vi "Authenticate.vi"(8 "error in (no error)":errorcluster, 10 "Authentication Inputs":T2, 11 "Authentication Provider in":refnum<class "Authentication Provider.lvclass">) -> (0 "error out":errorcluster, 2 "Authentication Outputs":T1, 3 "Authentication Provider out":refnum<class "Authentication Provider.lvclass">)   [LabVIEW 2020, in "HTTP Server.lvlib" / "Authentication Provider.lvclass"]
uses:
  Authentication Provider.lvclass
  Session/Session.lvclass
  lv-http-util/HTTP Utils/Request/Request.lvclass
  User Provider/User Provider.lvclass
  Authentication Inputs.ctl
  HTTP Server.lvlib
  User/User.lvclass
  Authentication Outputs.ctl
  Password Encoder/Password Encoder.lvclass
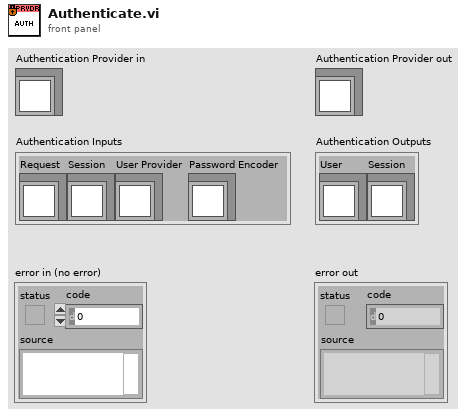
[diagram p1: front panel]
types:
  T1 = typedef "HTTP Server.lvlib/Authentication Outputs.ctl" = cluster{"User":refnum<class "User.lvclass">, "Session":refnum<class "Session.lvclass">}
  T2 = typedef "HTTP Server.lvlib/Authentication Inputs.ctl" = cluster{"Request":refnum<class "Request.lvclass">, "Session":refnum<class "Session.lvclass">, "User Provider":refnum<class "User Provider.lvclass">, "Password Encoder":refnum<class "Password Encoder.lvclass">}
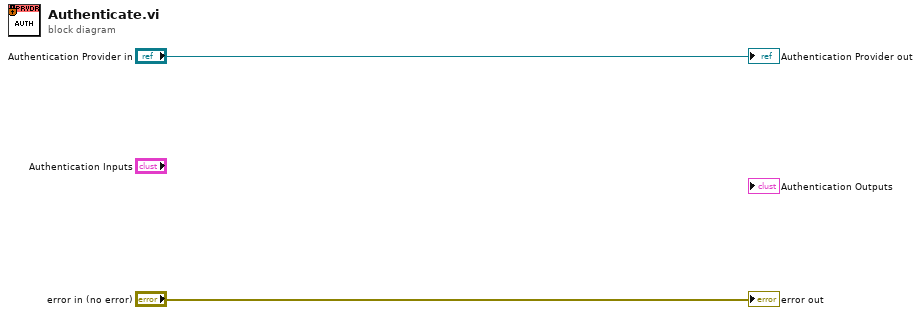
[diagram p0: block diagram]
diagram:
  "error out" <- "error in (no error)"
  "Authentication Provider out" <- "Authentication Provider in"
